vi "CMD_ROTATE.vi"(6 "Gantry in":refnum<class "Gantry.lvclass">, 8 "error in (no error)":errorcluster, 10 "Arguments":string[](array[string]), 11 "gScript Interpreter in":refnum<class "gScript Interpreter.lvclass">) -> (0 "error out":errorcluster, 3 "gScript Interpreter out":refnum<class "gScript Interpreter.lvclass">, 4 "Gantry out":refnum<class "Gantry.lvclass">)   [LabVIEW 2017, in "gScript Interpreter.lvclass"]
uses:
  gScript Interpreter.lvclass
  Shared Components/Gantry Class/Gantry.lvclass
  Shared Components/Orient3d Class/Orient3d.lvclass
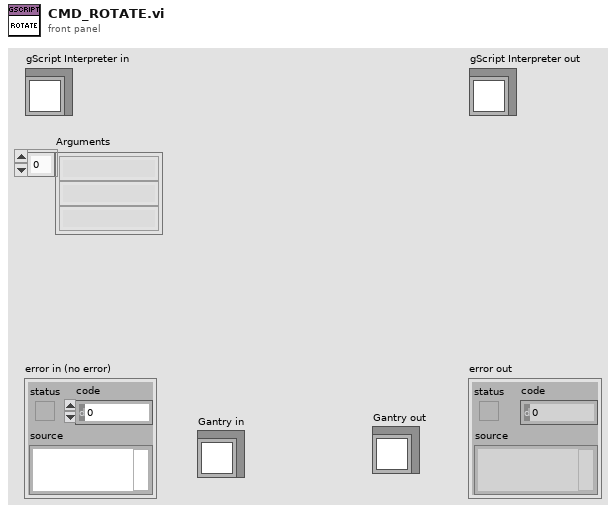
[diagram p1: front panel]
types:
  T1 = typedef "Memory Cell.ctl" = cluster{"type":T2, "x":dbl, "y":dbl, "z":dbl, "w":dbl}
  T2 = typedef "Memory Cell Type Enum.ctl" = enum16{"integer", "float", "vector", "rotation"}
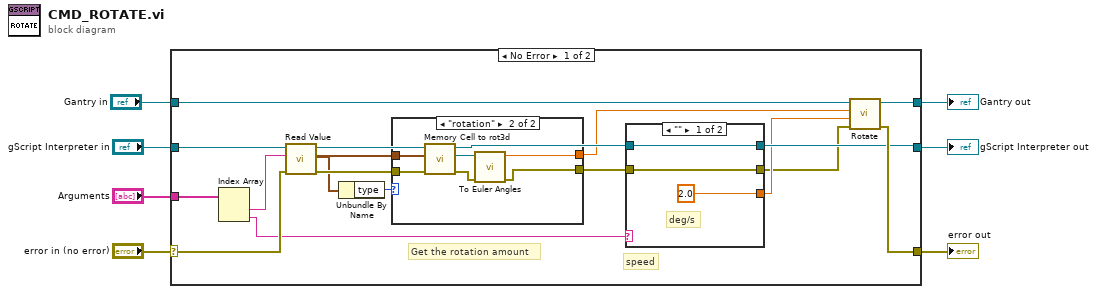
[diagram p0: block diagram]
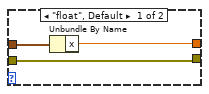
[diagram p2: hidden frame]
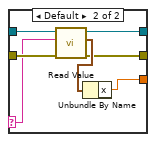
[diagram p3: hidden frame]
diagram:
  n1 = case shown="No Error" "error in (no error)" {
    selector: "error in (no error)" -> [w19 w45]
    tunnel: [w18 w45] -> w6
    tunnel: [w15 w44] -> w4
    tunnel: "gScript Interpreter in" -> [w22 w44]
    tunnel: "Arguments" -> [w21 _]
    tunnel: "Gantry in" -> [w24 w43]
    tunnel: [w23 w43] -> w1
    frame No Error {
      # "speed"
      # "Get the rotation amount"
      n2 = Index Array(array=w21) -> (element #1=w20:string, element #2=w17:string)  [unwired: 2 in]
      n3 = call-dynamic "Read Value.vi"("error in (no error)"=w19, "String in"=w20, "gScript Interpreter in"=w22) -> ("error out"=w11:errorcluster, "Memory Cell"=w10:T1, "gScript Interpreter out"=w16:refnum<class "gScript Interpreter.lvclass">)  [unwired: 6 in]
      n4 = Unbundle By Name(w10) -> ("type"=w12:T2)
      n5 = case shown="\"rotation\"" w12 {
        tunnel: w10 -> [w27 w32]
        tunnel: [w26 w30] -> w9
        tunnel: w11 -> [w25 w29]
        tunnel: [w25 w28] -> w8
        frame "float", Default {
          n6 = Unbundle By Name(w27) -> ("x"=w26:dbl)
        }
        frame "rotation" {
          n7 = call "Memory Cell to rot3d.vi"("Memory Cell"=w32) -> ("Orient3d out"=w31:refnum<class "Orient3d.lvclass">)  [unwired: 10 in]
          n8 = call "To Euler Angles.vi"("error in"=w29, "Orient3d in"=w31) -> ("error out"=w28:errorcluster, "psi/yaw"=w30:dbl)  [unwired: 6 in, 2 out]
        }
      }
      n9 = case shown="\"\"" w17 {
        selector: w17 -> [_ w39]
        tunnel: w16 -> [w35 w42]
        tunnel: w8 -> [w34 w41]
        tunnel: [w35 w40] -> w15
        tunnel: [w34 w37] -> w13
        tunnel: [2.0 w36] -> w14
        frame "" {
          # "deg/s"
        }
        frame Default {
          n10 = call-dynamic "Read Value.vi"("error in (no error)"=w41, "String in"=w39, "gScript Interpreter in"=w42) -> ("error out"=w37:errorcluster, "Memory Cell"=w38:T1, "gScript Interpreter out"=w40:refnum<class "gScript Interpreter.lvclass">)  [unwired: 6 in]
          n11 = Unbundle By Name(w38) -> ("x"=w36:dbl)
        }
      }
      n12 = call-dynamic "Rotate.vi"("error in"=w13, "speed(deg/s)"=w14, "distance(deg)"=w9, "Gantry in"=w24) -> ("error out"=w18:errorcluster, "Gantry out"=w23:refnum<class "Gantry.lvclass">)  [unwired: 6 in]
    }
    frame Error {
    }
  }
  "error out" <- w6
  "gScript Interpreter out" <- w4
  "Gantry out" <- w1
